vi "week04_Ex01.vi"() -> ()   [LabVIEW 2017]
panel:
  out "a?":bool
  out "concatenated string":string
  out "all lower case string 2":string
  out "all lower case string":string
  out "substring 2":string
  out "substring":string
  out "length":i32
  out "trimmed string":string
  out "Sting length":i32
  in  "String input":string
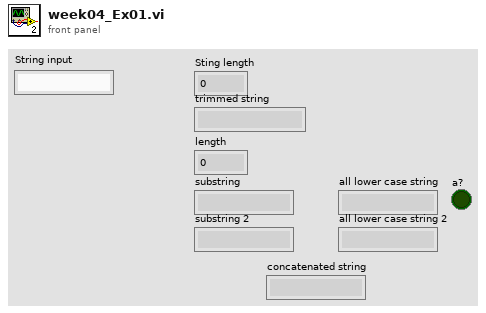
[diagram p1: front panel]
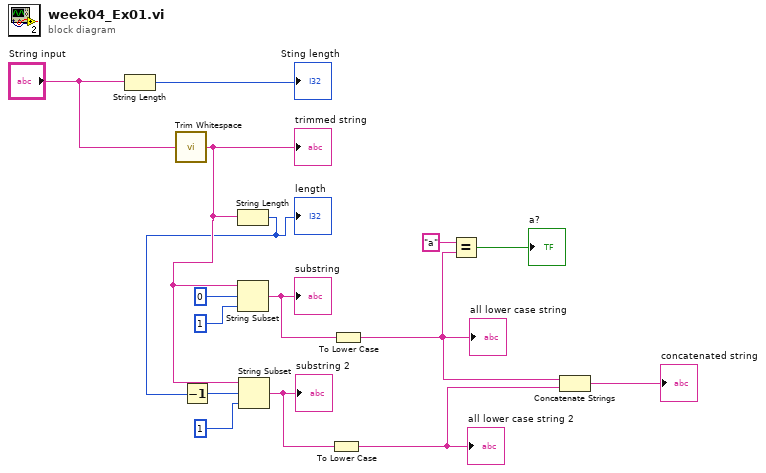
[diagram p0: block diagram]
diagram:
  n1 = String Length(string="String input") -> (length=→"Sting length":i32)
  n2 = call <vilib>:"Trim Whitespace.vi"("string"="String input") -> ("trimmed string"=w10:string)  [unwired: 1 in]
  "trimmed string" <- w10
  n3 = String Length(string=w10) -> (length=w8:i32)
  "length" <- w8
  n4 = Decrement(x=w8) -> (x-1=w9:i32)
  n5 = String Subset(string=w10, offset (0)=0, length (rest)=1 ("length (rest)")) -> (substring=w7:string)
  "substring" <- w7
  n6 = String Subset(string=w10, offset (0)=w9, length (rest)=1 ("length (rest)")) -> (substring=w6:string)
  "substring 2" <- w6
  n7 = To Lower Case(string=w6) -> (all lower case string=w5:string)
  "all lower case string 2" <- w5
  n8 = To Lower Case(string=w7) -> (all lower case string=w3:string)
  "all lower case string" <- w3
  n9 = Equal?(x="a", y=w3) -> (x = y?=→"a?":bool)
  n10 = Concatenate Strings(w3, w5) -> (→"concatenated string":string)
